vi "ToPythonVersionString_Namedtuples.vi"(11 "python version":T1) -> (3 "python version string":string)   [LabVIEW 2023]
doc: "Helper VI to convert from the Python version enum to a version string that is the input to the Open Python Session node."
uses:
  PythonVersionsEnum_Namedtuples.ctl
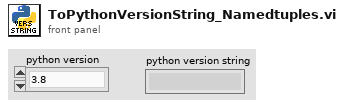
[diagram p1: front panel]
types:
  T1 = typedef "PythonVersionsEnum_Namedtuples.ctl" = enum16{"3.8", "3.9", "3.10"}
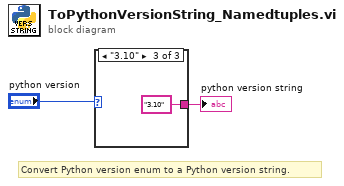
[diagram p0: block diagram]
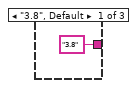
[diagram p2: hidden frame]
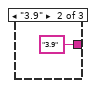
[diagram p3: hidden frame]
diagram:
  # "Convert Python version enum to a Python version string."
  n1 = case shown="\"3.10\"" "python version" {
    tunnel: ["3.8" ("python version") "3.9" ("python version") "3.10" ("python version")] -> w2
    frame "3.8", Default {
    }
    frame "3.9" {
    }
    frame "3.10" {
    }
  }
  "python version string" <- w2
